vi "Update U16.vi"(6 "Image Array Dims":cluster{"Shots":dbl, "Height":dbl, "Width":dbl}, 8 "error in (no error)":errorcluster, 9 "Image Series":u16[](array[numeric]), 10 "Analysis Image":dbl[][](array[numeric]), 11 "Analysis Graph in":refnum<class "Analysis Graph.lvclass">) -> (0 "error out":errorcluster, 1 "pixel signal roied  out":u16[](array[numeric]), 2 "Cursor.Cursor Position":T1, 3 "Analysis Graph out":refnum<class "Analysis Graph.lvclass">)   [LabVIEW 2023]
uses:
  Analysis Graph.lvclass
  <vilib>/Utility/miscctls.llb/LVPointDoubleTypeDef.ctl
  Series Graph/Series Graph.lvclass/Series Graph.ctl
  Detail Graph/Detail Graph.lvclass
  Series Graph/Series Graph.lvclass
  D:/git/Graph-Classes/graph-classes/Series Graph/Series Graph.lvclass
  D:/git/Graph-Classes/graph-classes/Detail Graph/Detail Graph.lvclass
  D:/git/Graph-Classes/graph-classes/Base Graph/Base Graph.lvclass
  D:/git/Graph-Classes/graph-classes/Analysis Graph/Analysis Graph.lvclass
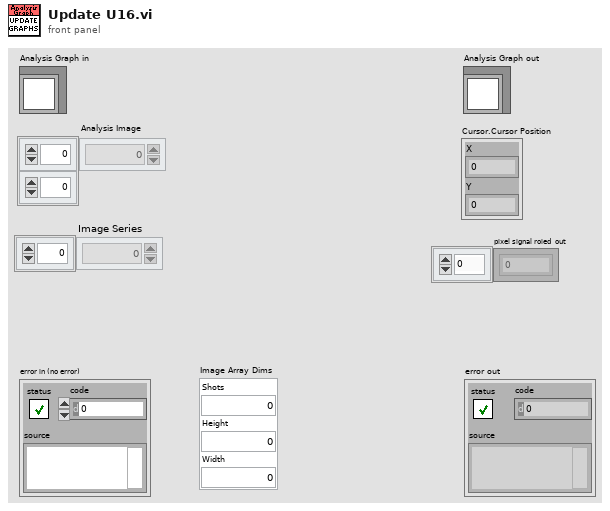
[diagram p1: front panel]
types:
  T1 = typedef "LVPointDoubleTypeDef.ctl" = cluster{"X":dbl, "Y":dbl}
  T2 = cluster{"ROI X":cluster{"Index":u32, "Length":u32}, "ROI Y":cluster{"Index":u32, "Length":u32}, "ROI Z":cluster{"Index":u32, "Length":u32}}
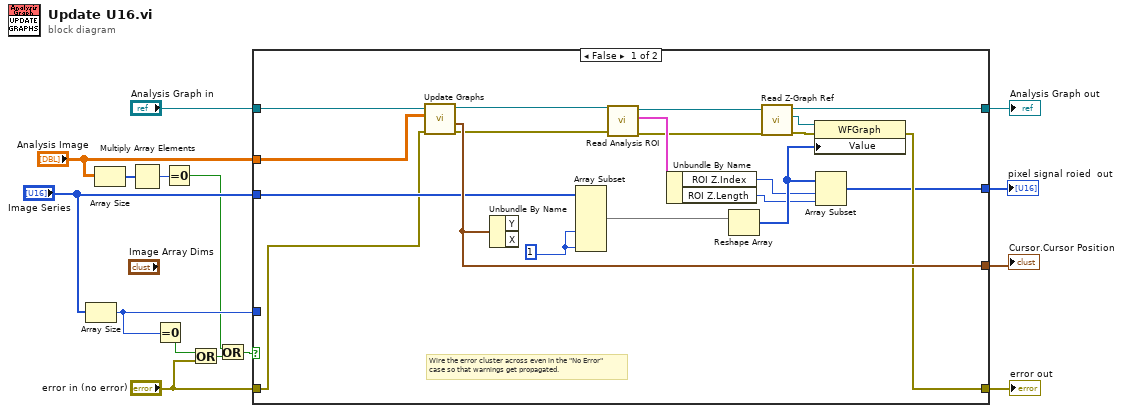
[diagram p0: block diagram]
diagram:
  n1 = Array Size(array="Image Series") -> (size(s)=w10:i32)
  n2 = Array Size(array="Analysis Image") -> (size(s)=w5:i32[])
  n3 = Multiply Array Elements(1:w5) -> (0:w4:i32)
  n4 = Equal To 0?(x=w10) -> (x = 0?=w12:bool)
  n5 = Equal To 0?(x=w4) -> (x = 0?=w3:bool)
  n6 = Or(x=w12, y="error in (no error)") -> (x .or. y?=w2:bool)
  n7 = Or(x=w3, y=w2) -> (x .or. y?=w1:bool)
  n8 = case shown="False" w1 {
    tunnel: [w30 w37] -> w15
    tunnel: [w35 w38] -> w13
    tunnel: "Analysis Graph in" -> [w23 w38]
    tunnel: "error in (no error)" -> [w22 w37]
    tunnel: w10 -> [_ _]
    tunnel: "Analysis Image" -> [w32 _]
    tunnel: "Image Series" -> [w29 _]
    tunnel: [w31 _] -> w8
    tunnel: [w16 _] -> w7
    frame False {
      w36 = 1 ("length")
      # "Wire the error cluster across even in the \"No Error\"\ncase so that warnings get propagated."
      n9 = call "Update Graphs.vi"("error in (no error)"=w22, "image"=w32, "Detail Graph in"=w23) -> ("error out"=w25:errorcluster, "Cursor.Cursor Position"=w31:T1, "Detail Graph out"=w21:refnum<class "Analysis Graph.lvclass">)  [unwired: 6 in]
      n10 = Unbundle By Name(w31) -> ()  [unwired: 2 out]
      n11 = Array Subset(array=w29, length (dim 1)=w36, length (dim 2)=w36) -> (w27:u16[])  [unwired: 4 in]
      n12 = call "Read Analysis ROI.vi"("error in (no error)"=w25, "Analysis Graph in"=w21) -> ("error out"=w24:errorcluster, "ROI XYZ"=w26:T2, "Analysis Graph out"=w20:refnum<class "Analysis Graph.lvclass">)  [unwired: 7 in]
      n13 = Unbundle By Name(w26) -> ("ROI Z.Index"=w18:u32, "ROI Z.Length"=w17:u32)
      n14 = Reshape Array(w27) -> (w19:u16[], w28:i32)
      n15 = call "Read Z-Graph Ref.vi"("error in (no error)"=w24, "Series Graph in"=w20) -> ("error out"=w33:errorcluster, "Z-Graph Ref"=w34:refnum<vi>, "Series Graph out"=w35:refnum<class "Analysis Graph.lvclass">)  [unwired: 7 in]
      n16 = property class="WFGraph"(reference=w34, error in=w33, "Value"=w19) -> (error out=w30:errorcluster)  [unwired: 1 out]
      n17 = Array Subset(array=w19, index=w18, length=w17) -> (w16:u16[])
    }
    frame True {
    }
  }
  "error out" <- w15
  "Analysis Graph out" <- w13
  "Cursor.Cursor Position" <- w8
  "pixel signal roied  out" <- w7
